vi "MassFlow to Velocity.vi"(9 "Mass Flow (kg/s)":dbl, 10 "Density (kg/m^3)":dbl, 11 "Area (m^2)":dbl) -> (3 "Velocity (m/s)":dbl)   [LabVIEW 2019]
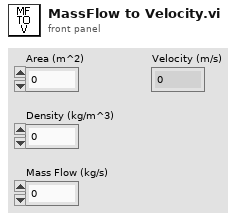
[diagram p1: front panel]
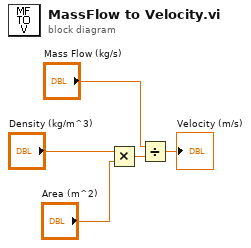
[diagram p0: block diagram]
diagram:
  n1 = Multiply(x="Density (kg/m^3)", y="Area (m^2)") -> (x*y=w4:dbl)
  n2 = Divide(x="Mass Flow (kg/s)", y=w4) -> (x/y=→"Velocity (m/s)":dbl)
